vi "Write DMA.vi"(8 "error in (no error)":errorcluster, 10 "Refs":T3={"Data Type"=enum."I32", "DMA_SGL"=refnum, "DMA_U64"=refnum, "DMA_I64"=refnum, "DMA_FXP+/-32.8"=refnum, "DMA_FXP+/-64.32"=refnum, "DMA_U32"=refnum, "DMA_U16"=refnum, "DMA_U8"=refnum, "DMA_I32"=refnum, "DMA_I16"=refnum, "DMA_I8"=refnum, "DMA_FXP+/-32.16"=refnum} {"Data Type" format="%.0x"}, 11 "Waveform Refs":refnum<class "Single Waveform Read (DBL).lvclass">[](array[class])) -> (0 "error out":errorcluster, 1 "Empty Elements Remaining":u32, 2 "Refs out":T3={"Data Type"=enum."I32", "DMA_SGL"=refnum, "DMA_U64"=refnum, "DMA_I64"=refnum, "DMA_FXP+/-32.8"=refnum, "DMA_FXP+/-64.32"=refnum, "DMA_U32"=refnum, "DMA_U16"=refnum, "DMA_U8"=refnum, "DMA_I32"=refnum, "DMA_I16"=refnum, "DMA_I8"=refnum, "DMA_FXP+/-32.16"=refnum} {"Data Type" format="%.0x"}, 3 "Waveform Refs":refnum<class "Single Waveform Read (DBL).lvclass">[](array[class]), 4 "Wafeform Properties":T1[](array[typedef]))   [LabVIEW 2020, in "FPGA Addon Engine.lvlib"]
uses:
  FPGA Addon Engine.lvlib
  Types/DMA Output Refs.ctl
  Addon Shared/Types/FPGA Addon Data Type.ctl
  <vilib>/NI VeriStand/Custom Device Waveform API/Single Waveform Read (DBL)/Single Waveform Read (DBL).lvclass
  C:/Program Files (x86)/National Instruments/LabVIEW 2020/vi.lib/NI VeriStand/Custom Device Waveform API/Waveform Session.lvclass
  <vilib>/NI VeriStand/Custom Device Waveform API/Waveform Session.lvclass/Waveform Session.ctl
  <vilib>/NI VeriStand/Custom Device Waveform API/Single Waveform Read (DBL)/Single Waveform Read (DBL).lvclass/Single Waveform Read (DBL).ctl
  <vilib>/NI VeriStand/Custom Device Waveform API/Internal Comm Classes/WPL Comm/WPL Comm (1D DBL)/WPL Comm (1D DBL).lvclass/WPL Comm (1D DBL).ctl
  <vilib>/NI VeriStand/Custom Device Waveform API/Internal Comm Classes/WPL Comm/WPL Comm (1D DBL)/Comm_read 1d dbl.vi
  <vilib>/NI VeriStand/Custom Device Waveform API/Check Opened.vi
  <vilib>/NI VeriStand/Custom Device Waveform API/Internal Comm Classes/WPL Comm/Convert Q Error to Shutdown Error.vi
  <vilib>/Utility/error.llb/Error Cluster From Error Code.vi
  <vilib>/rvi/errors/niLvFpgaAdjustHostInterfaceError.vi
  <vilib>/rvi/interface/nirviMethod/nirviMethod.xnode
  <vilib>/NI VeriStand/Custom Device Waveform API/Single Waveform Read (DBL)/NI VeriStand - Read Single Waveform (DBL).vi
  <vilib>/NI VeriStand/Custom Device Waveform API/NI_VS Custom Device Waveform API.lvlib
  <vilib>/FPGAPlugInAG/Dynamic/niLvFpga_WriteFifo_Dynamic.vi
  <vilib>/rvi/errors/niLvFpgaMergeErrorWithErrorCode.vi
  Addon Shared/FPGA Addon Shared.lvlib
  <vilib>/NI VeriStand/Custom Device API/Waveform Data Reference.ctl
  <vilib>/NI VeriStand/Custom Device API/Custom Device API.lvlib
  <vilib>/NI VeriStand/Custom Device Waveform API/Waveform properties.ctl
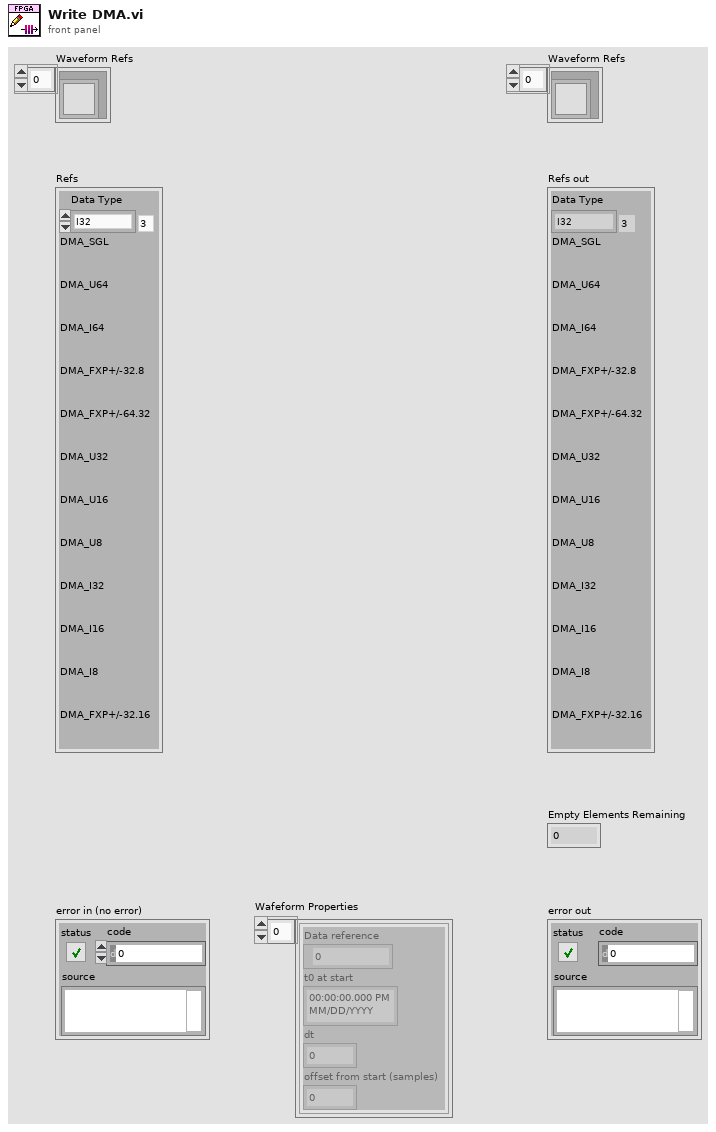
[diagram p1: front panel]
types:
  T1 = typedef "NI_VS Custom Device Waveform API.lvlib/Waveform properties.ctl" = cluster{"Data reference":T2, "t0 at start":timestamp, "dt":dbl, "offset from start (samples)":u64}
  T2 = typedef "Custom Device API.lvlib/Waveform Data Reference.ctl" = i32
  T3 = typedef "FPGA Addon Engine.lvlib/DMA Output Refs.ctl" = cluster{"Data Type":T4, "DMA_SGL":refnum<k20>, "DMA_U64":refnum<k20>, "DMA_I64":refnum<k20>, "DMA_FXP+/-32.8":refnum<k20>, "DMA_FXP+/-64.32":refnum<k20>, "DMA_U32":refnum<k20>, "DMA_U16":refnum<k20>, "DMA_U8":refnum<k20>, "DMA_I32":refnum<k20>, "DMA_I16":refnum<k20>, "DMA_I8":refnum<k20>, "DMA_FXP+/-32.16":refnum<k20>}
  T4 = typedef "FPGA Addon Shared.lvlib/FPGA Addon Data Type.ctl" = enum8{"<Null>", "I8", "I16", "I32", "I64", "U8", "U16", "U32", "U64", "SGL", "Boolean", "Analog PWM In Settings", "Analog PWM In", "Digital PWM In Settings", "Digital PWM In", "Digital PWM Out", "Sine Out", "FXP", "FXP+/-24.5", "FXP+/-16.5", "FXP+/-32.8", "FXP+/-64.32", "FXP+/-16.7", "FXP+/-20.5", "FXP+/-27.5", "FXP+/-32.16", "FXP+16.3", "FXP+18.3", "Digital Static In", "Digital Static Out", "Digital Static In Settings", "Digital WSS Out", "Quad Encoder Settings", "Quad Encoder In", "Group"}
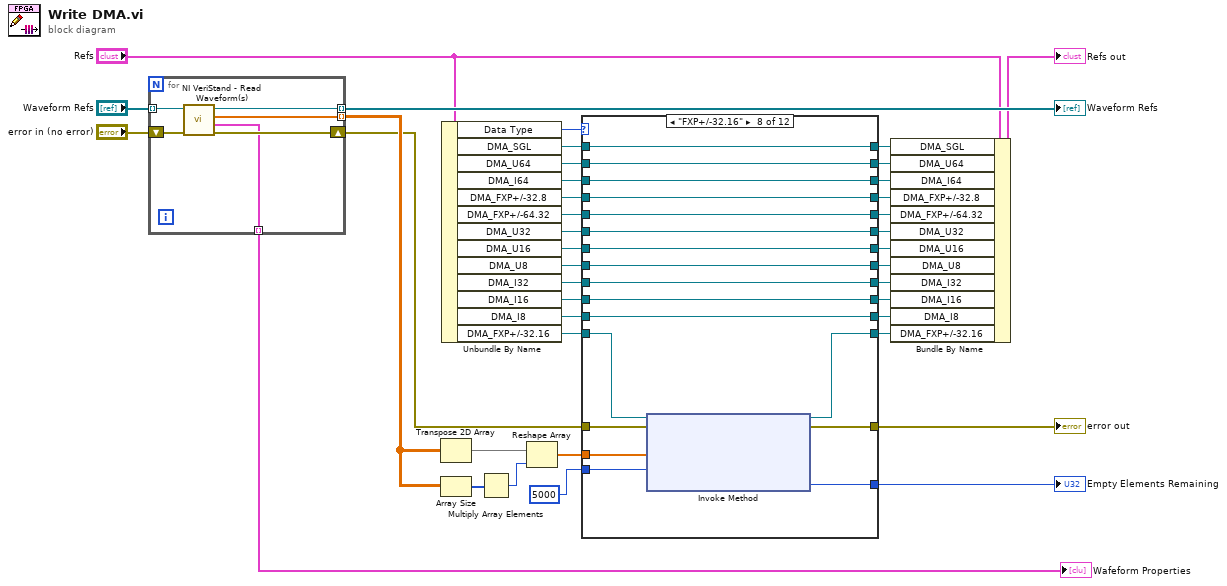
[diagram p0: block diagram]
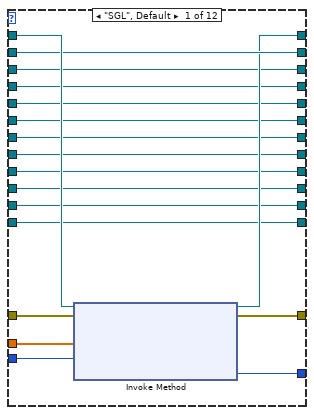
[diagram p2: hidden frame]
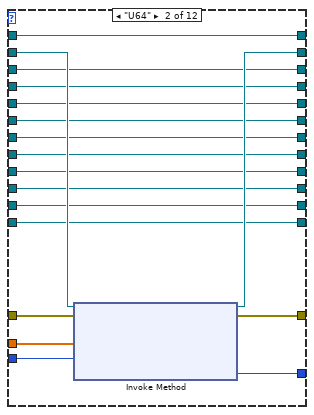
[diagram p3: hidden frame]
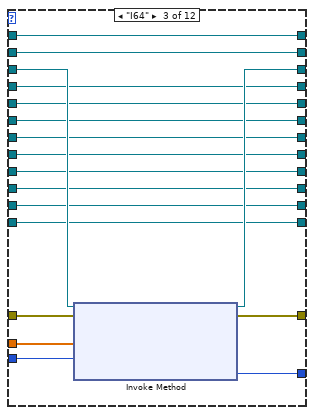
[diagram p4: hidden frame]
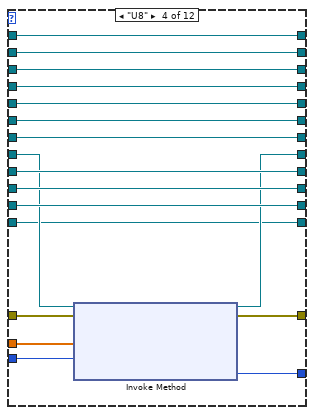
[diagram p5: hidden frame]
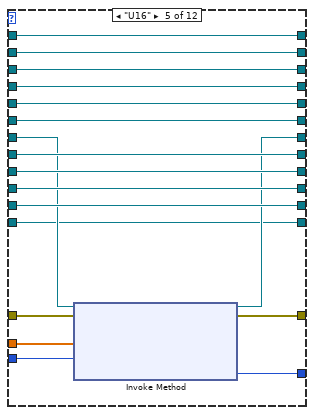
[diagram p6: hidden frame]
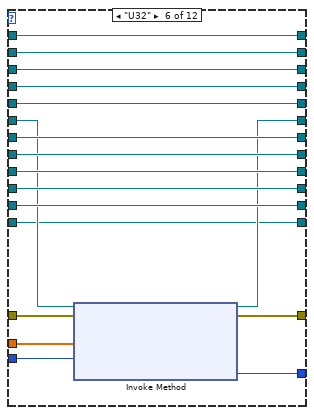
[diagram p7: hidden frame]
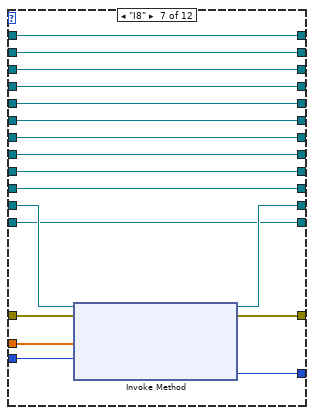
[diagram p8: hidden frame]
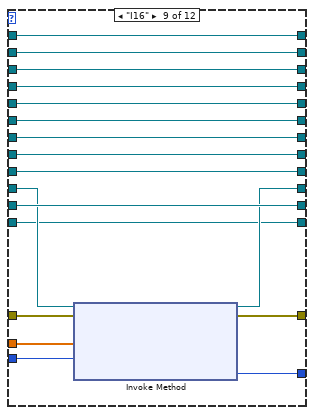
[diagram p9: hidden frame]
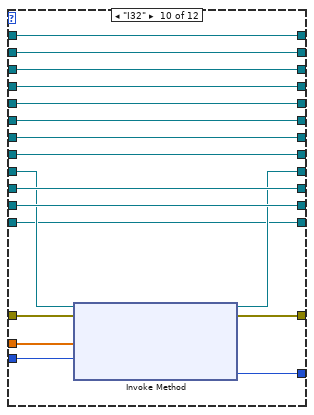
[diagram p10: hidden frame]
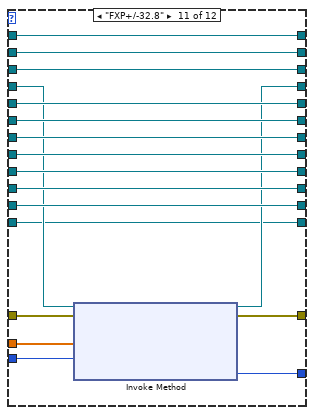
[diagram p11: hidden frame]
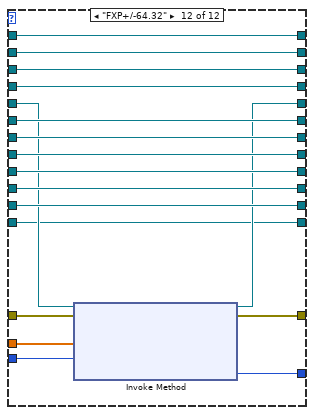
[diagram p12: hidden frame]
diagram:
  n1 = for {
    tunnel: [w46] -> w30 mode=indexing
    shift-right: [w45] -> w29
    shift-left: "error in (no error)" -> [w44]
    tunnel: "Waveform Refs" -> [w43] mode=indexing
    tunnel: [w42] -> w35 mode=indexing
    tunnel: [w41] -> w1 mode=indexing
    n2 = call-poly <vilib>:"NI VeriStand - Read Waveform(s).vi"("error in (no error)"=w44, "Single Waveform Read Session (DBL) in"=w43) -> ("error out"=w45:errorcluster, "Properties"=w41:T1, "Data"=w46:dbl[], "Single Waveform Read Session (DBL) out"=w42:refnum<class "Single Waveform Read (DBL).lvclass">)  [unwired: 5 in, 1 out]
  }
  "Waveform Refs" <- w35
  "Wafeform Properties" <- w1
  n3 = Transpose 2D Array(2D array=w30) -> (transposed array=w31:dbl[][])
  n4 = Array Size(array=w30) -> (size(s)=w33:i32[])
  n5 = Unbundle By Name("Refs") -> ("Data Type"=w28:T4, "DMA_SGL"=w27:refnum<k20>, "DMA_U64"=w26:refnum<k20>, "DMA_I64"=w21:refnum<k20>, "DMA_FXP+/-32.8"=w18:refnum<k20>, "DMA_FXP+/-64.32"=w16:refnum<k20>, "DMA_U32"=w14:refnum<k20>, "DMA_U16"=w12:refnum<k20>, "DMA_U8"=w10:refnum<k20>, "DMA_I32"=w8:refnum<k20>, "DMA_I16"=w6:refnum<k20>, "DMA_I8"=w4:refnum<k20>, "DMA_FXP+/-32.16"=w3:refnum<k20>)
  n6 = Multiply Array Elements(1:w33) -> (0:w32:i32)
  n7 = Reshape Array(w31, w32) -> (w37:dbl[])
  n8 = case shown="\"FXP+/-32.16\"" w28 {
    tunnel: [w64 w82 w100 w118 w136 w154 w172 w190 w208 w226 w244 w262] -> w40
    tunnel: [w63 w81 w99 w117 w135 w153 w171 w189 w207 w225 w243 w261] -> w39
    tunnel: 5000 ("Timeout (ms)") -> [w62 w80 w98 w116 w134 w152 w170 w188 w206 w224 w242 w260]
    tunnel: w37 -> [w61 w79 w97 w115 w133 w151 w169 w187 w205 w223 w241 w259]
    tunnel: w29 -> [w60 w78 w96 w114 w132 w150 w168 w186 w204 w222 w240 w258]
    tunnel: w27 -> [w59 w77 w95 w113 w131 w149 w167 w185 w203 w221 w239 w257]
    tunnel: [w58 w75 w92 w112 w130 w148 w166 w184 w202 w220 w238 w256] -> w24
    tunnel: w26 -> [w58 w76 w92 w112 w130 w148 w166 w184 w202 w220 w238 w256]
    tunnel: [w57 w77 w95 w113 w131 w149 w167 w185 w203 w221 w239 w257] -> w23
    tunnel: w21 -> [w56 w74 w94 w104 w122 w140 w158 w176 w194 w212 w230 w248]
    tunnel: [w56 w74 w93 w104 w122 w140 w158 w176 w194 w212 w230 w248] -> w20
    tunnel: [w48 w66 w91 w111 w129 w147 w165 w183 w201 w219 w228 w255] -> w19
    tunnel: w18 -> [w48 w66 w91 w111 w129 w147 w165 w183 w201 w219 w229 w255]
    tunnel: [w49 w67 w90 w110 w128 w146 w164 w182 w200 w218 w237 w246] -> w17
    tunnel: w16 -> [w49 w67 w90 w110 w128 w146 w164 w182 w200 w218 w237 w247]
    tunnel: [w50 w68 w89 w109 w127 w138 w163 w181 w199 w217 w236 w254] -> w15
    tunnel: w14 -> [w50 w68 w89 w109 w127 w139 w163 w181 w199 w217 w236 w254]
    tunnel: [w51 w69 w88 w108 w120 w145 w162 w180 w198 w216 w235 w253] -> w13
    tunnel: w12 -> [w51 w69 w88 w108 w121 w145 w162 w180 w198 w216 w235 w253]
    tunnel: [w52 w70 w87 w102 w126 w144 w161 w179 w197 w215 w234 w252] -> w11
    tunnel: w10 -> [w52 w70 w87 w103 w126 w144 w161 w179 w197 w215 w234 w252]
    tunnel: [w53 w71 w86 w107 w125 w143 w160 w178 w196 w210 w233 w251] -> w9
    tunnel: w8 -> [w53 w71 w86 w107 w125 w143 w160 w178 w196 w211 w233 w251]
    tunnel: [w54 w72 w85 w106 w124 w142 w159 w177 w192 w214 w232 w250] -> w7
    tunnel: w6 -> [w54 w72 w85 w106 w124 w142 w159 w177 w193 w214 w232 w250]
    tunnel: [w55 w73 w84 w105 w123 w141 w156 w173 w195 w213 w231 w249] -> w5
    tunnel: w4 -> [w55 w73 w84 w105 w123 w141 w157 w173 w195 w213 w231 w249]
    tunnel: w3 -> [w47 w65 w83 w101 w119 w137 w155 w175 w191 w209 w227 w245]
    tunnel: [w47 w65 w83 w101 w119 w137 w155 w174 w191 w209 w227 w245] -> w2
    frame "SGL", Default {
      n9 = xnode "Invoke Method"("FPGA VI Reference In"=w59, "error in"=w60, "Data"=w61, "Timeout (ms)"=w62) -> ("FPGA VI Reference Out"=w57:refnum<k20>, "error out"=w64:errorcluster, "Empty Elements Remaining"=w63:u32)
    }
    frame "U64" {
      n10 = xnode "Invoke Method"("FPGA VI Reference In"=w76, "error in"=w78, "Data"=w79, "Timeout (ms)"=w80) -> ("FPGA VI Reference Out"=w75:refnum<k20>, "error out"=w82:errorcluster, "Empty Elements Remaining"=w81:u32)
    }
    frame "I64" {
      n11 = xnode "Invoke Method"("FPGA VI Reference In"=w94, "error in"=w96, "Data"=w97, "Timeout (ms)"=w98) -> ("FPGA VI Reference Out"=w93:refnum<k20>, "error out"=w100:errorcluster, "Empty Elements Remaining"=w99:u32)
    }
    frame "U8" {
      n12 = xnode "Invoke Method"("FPGA VI Reference In"=w103, "error in"=w114, "Data"=w115, "Timeout (ms)"=w116) -> ("FPGA VI Reference Out"=w102:refnum<k20>, "error out"=w118:errorcluster, "Empty Elements Remaining"=w117:u32)
    }
    frame "U16" {
      n13 = xnode "Invoke Method"("FPGA VI Reference In"=w121, "error in"=w132, "Data"=w133, "Timeout (ms)"=w134) -> ("FPGA VI Reference Out"=w120:refnum<k20>, "error out"=w136:errorcluster, "Empty Elements Remaining"=w135:u32)
    }
    frame "U32" {
      n14 = xnode "Invoke Method"("FPGA VI Reference In"=w139, "error in"=w150, "Data"=w151, "Timeout (ms)"=w152) -> ("FPGA VI Reference Out"=w138:refnum<k20>, "error out"=w154:errorcluster, "Empty Elements Remaining"=w153:u32)
    }
    frame "I8" {
      n15 = xnode "Invoke Method"("FPGA VI Reference In"=w157, "error in"=w168, "Data"=w169, "Timeout (ms)"=w170) -> ("FPGA VI Reference Out"=w156:refnum<k20>, "error out"=w172:errorcluster, "Empty Elements Remaining"=w171:u32)
    }
    frame "FXP+/-32.16" {
      n16 = xnode "Invoke Method"("FPGA VI Reference In"=w175, "error in"=w186, "Data"=w187, "Timeout (ms)"=w188) -> ("FPGA VI Reference Out"=w174:refnum<k20>, "error out"=w190:errorcluster, "Empty Elements Remaining"=w189:u32)
    }
    frame "I16" {
      n17 = xnode "Invoke Method"("FPGA VI Reference In"=w193, "error in"=w204, "Data"=w205, "Timeout (ms)"=w206) -> ("FPGA VI Reference Out"=w192:refnum<k20>, "error out"=w208:errorcluster, "Empty Elements Remaining"=w207:u32)
    }
    frame "I32" {
      n18 = xnode "Invoke Method"("FPGA VI Reference In"=w211, "error in"=w222, "Data"=w223, "Timeout (ms)"=w224) -> ("FPGA VI Reference Out"=w210:refnum<k20>, "error out"=w226:errorcluster, "Empty Elements Remaining"=w225:u32)
    }
    frame "FXP+/-32.8" {
      n19 = xnode "Invoke Method"("FPGA VI Reference In"=w229, "error in"=w240, "Data"=w241, "Timeout (ms)"=w242) -> ("FPGA VI Reference Out"=w228:refnum<k20>, "error out"=w244:errorcluster, "Empty Elements Remaining"=w243:u32)
    }
    frame "FXP+/-64.32" {
      n20 = xnode "Invoke Method"("FPGA VI Reference In"=w247, "error in"=w258, "Data"=w259, "Timeout (ms)"=w260) -> ("FPGA VI Reference Out"=w246:refnum<k20>, "error out"=w262:errorcluster, "Empty Elements Remaining"=w261:u32)
    }
  }
  "error out" <- w40
  "Empty Elements Remaining" <- w39
  n21 = Bundle By Name(cluster="Refs", "DMA_SGL"=w23, "DMA_U64"=w24, "DMA_I64"=w20, "DMA_FXP+/-32.8"=w19, "DMA_FXP+/-64.32"=w17, "DMA_U32"=w15, "DMA_U16"=w13, "DMA_U8"=w11, "DMA_I32"=w9, "DMA_I16"=w7, "DMA_I8"=w5, "DMA_FXP+/-32.16"=w2) -> (→"Refs out":T3)
